vi "CSTK_Enum_Creator_CreateTemporaryControlVI.vi"(8 "错误输入（无错误）":errorcluster) -> (0 "错误输出":errorcluster, 3 "VI输出":refnum<vi>)   [LabVIEW 2015, in "CSTK_Enum Creator.lvlib"]
uses:
  CSTK_Enum Creator.lvlib
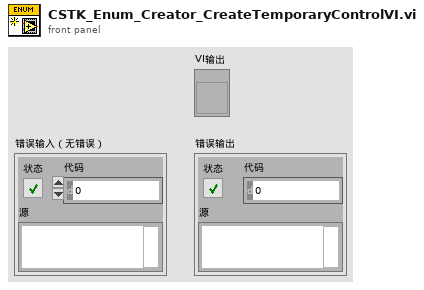
[diagram p1: front panel]
types:
  T1 = enum32{"invalid VI type", "Standard VI", "Control VI", "Global VI", "Polymorphic VI", "Configuration VI", "SubSystem", "Facade VI", "Method VI", "Statechart Diagram VI"}
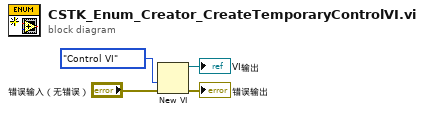
[diagram p0: block diagram]
diagram:
  n1 = New VI(8:"错误输入（无错误）", 9:T1."Control VI" ("VI类型（标准VI）")) -> (0:→"错误输出":errorcluster, 3:→"VI输出":refnum<vi>)  [unwired: 5 in]
